vi "Excel_Insert_Picture.vi"(5 "position fix":T1, 6 "name":string, 7 "Shapes":refnum<k7>, 8 "error in (no error)":errorcluster, 9 "position":cluster{"Left":i32, "Top":i32}, 10 "Filename":string, 11 "Worksheet":refnum<k7>) -> (0 "error out":errorcluster)   [LabVIEW 2015, in "NI_ReportGenerationToolkit.lvlib"]
uses:
  <vilib>/addons/_office/NI_ReportGenerationToolkit.lvlib
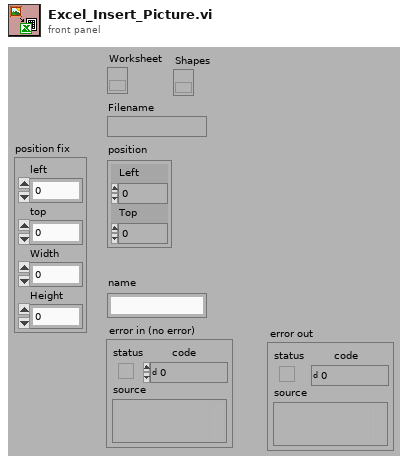
[diagram p1: front panel]
types:
  T1 = cluster{"left":dbl, "top":dbl, "Width":dbl, "Height":dbl}
  T2 = typedef "imagedata.ctl" = cluster{"image type":i32, "image depth":i32, "image":u8[], "mask":u8[], "colors":u32[], "Rectangle":cluster{"left":i16, "top":i16, "right":i16, "bottom":i16}}
  T3 = cluster{"left":i16, "top":i16, "right":i16, "bottom":i16}
  T4 = cluster{"left":dbl, "top":dbl, "right":dbl, "bottom":dbl}
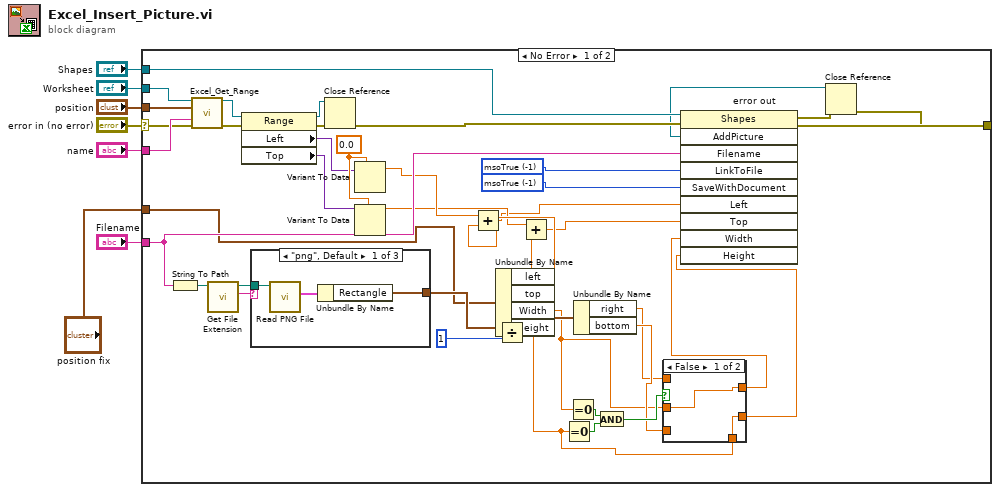
[diagram p0: block diagram]
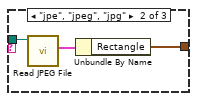
[diagram p3: hidden frame]
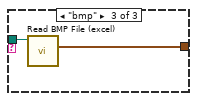
[diagram p4: hidden frame]
diagram:
  n1 = case shown="No Error" "error in (no error)" {
    selector: "error in (no error)" -> [w31 w62]
    tunnel: [w47 w62] -> w8
    tunnel: "Filename" -> [w41 _]
    tunnel: "Worksheet" -> [w34 _]
    tunnel: "name" -> [w33 _]
    tunnel: "position" -> [w32 _]
    tunnel: "Shapes" -> [w29 _]
    tunnel: "position fix" -> [w25 _]
    frame No Error {
      w44 = sgl 0.0 ("Left")
      w48 = -1 items=["msoTrue"=-1, "msoFalse"=0, "msoCTrue"=1, "msoTriStateToggle"=-3, "msoTriStateMixed"=-2] ("LinkToFile")
      w49 = -1 items=["msoTrue"=-1, "msoFalse"=0, "msoCTrue"=1, "msoTriStateToggle"=-3, "msoTriStateMixed"=-2] ("SaveWithDocument")
      n2 = String To Path(string=w41) -> (path=w28:path)
      n3 = call <vilib>:"Excel_Get_Range.vi"("Excel._Worksheet"=w34, "start"=w32, "name"=w33, "error in (no error)"=w31) -> ("Range"=w30:refnum<k7>, "error out"=w35:errorcluster)  [unwired: 1 in, 9 out]
      n4 = call <vilib>:"Get File Extension.vi"("file"=w28) -> ("lowercase file extension"=w26:string, "dup file"=w27:path)  [unwired: 1 in, 8 out]
      n5 = property class="Range"(reference=w30, error in=w35) -> (reference out=w45:refnum<k7>, error out=w46:errorcluster, "Left"=w43:variant, "Top"=w42:variant)
      n6 = case shown="\"png\", Default" w26 {
        tunnel: w27 -> [w56 w59 w61]
        tunnel: [w54 w57 w60] -> w40
        frame "png", Default {
          n7 = call <vilib>:"Read PNG File.vi"("path to PNG file"=w56) -> ("image data"=w55:T2)  [unwired: 1 in, 9 out]
          n8 = Unbundle By Name(w55) -> ("Rectangle"=w54:T3)
        }
        frame "jpe", "jpeg", "jpg" {
          n9 = call <vilib>:"Read JPEG File.vi"("path to JPEG file"=w59) -> ("image data"=w58:T2)  [unwired: 1 in, 9 out]
          n10 = Unbundle By Name(w58) -> ("Rectangle"=w57:T3)
        }
        frame "bmp" {
          n11 = call <vilib>:"Read BMP File (excel).vi"("path to BMP file"=w61) -> ("rect"=w60:T3)  [unwired: 1 in, 9 out]
        }
      }
      n12 = Close Reference(reference=w45, error in (no error)=w46) -> (error out=w37:errorcluster)
      n13 = Variant To Data(type=w44, Variant=w43) -> (data=w23:sgl)  [unwired: 1 in, 1 out]
      n14 = Variant To Data(type=w44, Variant=w42) -> (data=w21:sgl)  [unwired: 1 in, 1 out]
      n15 = Unbundle By Name(w25) -> ("left"=w24:dbl, "top"=w22:dbl, "Width"=w10:dbl, "Height"=w9:dbl)
      n16 = Add(x=w23, y=w24) -> (x+y=w19:dbl)
      n17 = Divide(x=w40, y=1) -> (x/y=w38:T4)
      n18 = Add(x=w21, y=w22) -> (x+y=w20:dbl)
      n19 = Equal To 0?(x=w9) -> (x = 0?=w16:bool)
      n20 = Equal To 0?(x=w10) -> (x = 0?=w17:bool)
      n21 = Unbundle By Name(w38) -> ("right"=w11:dbl, "bottom"=w13:dbl)
      n22 = And(x=w17, y=w16) -> (x .and. y?=w15:bool)
      n23 = case shown="False" w15 {
        tunnel: [w50 w53] -> w14
        tunnel: w13 -> [_ w53]
        tunnel: [w51 w52] -> w12
        tunnel: w11 -> [_ w52]
        tunnel: w10 -> [w51 _]
        tunnel: w9 -> [w50 _]
        frame False {
        }
        frame True {
        }
      }
      n24 = invoke class="Shapes" method="AddPicture"(reference=w29, error in=w37, "Filename"=w41, "LinkToFile"=w48, "SaveWithDocument"=w49, "Left"=w19, "Top"=w20, "Width"=w12, "Height"=w14) -> (error out=w36:errorcluster, "AddPicture"=w18:refnum<k7>)  [unwired: 1 in, 8 out]
      n25 = Close Reference(reference=w18, error in (no error)=w36) -> (error out=w47:errorcluster)
    }
    frame Error {
    }
  }
  "error out" <- w8
